vi "Dequeue Message.vi"(8 "error in":errorcluster, 11 "module reference in":T1) -> (0 "error out":errorcluster, 1 "source":T2, 2 "data":variant, 3 "module reference out":T1, 5 "message":T5)   [LabVIEW 2017, in "Logger.lvlib"]
uses:
  Logger.lvlib
  Private TypeDefs/Messages.ctl
  Global TypeDefs/Registered Modules.ctl
  Private TypeDefs/Module Reference.ctl
  Private TypeDefs/Module Queues.ctl
  Private TypeDefs/Message Queue Element.ctl
  Private TypeDefs/Module Notifiers.ctl
  Private TypeDefs/Dummy Notifier.ctl
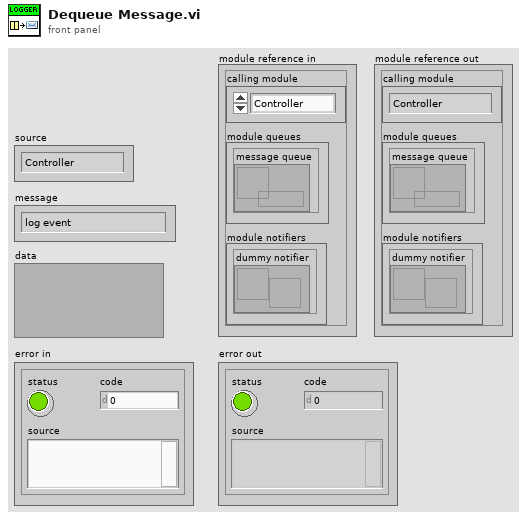
[diagram p1: front panel]
types:
  T1 = typedef "Logger.lvlib/Module Reference.ctl" = cluster{"calling module":T2, "module queues":T3, "module notifiers":T4}
  T2 = typedef "Registered Modules.ctl" = enum16{"Controller", "DAQ", "Error Handler", "Game", "myPAM", "WinHost", "Logger"}
  T3 = typedef "Logger.lvlib/Module Queues.ctl" = cluster{"message queue":refnum<queue>}
  T4 = typedef "Logger.lvlib/Module Notifiers.ctl" = cluster{"dummy notifier":refnum<notifier>}
  T5 = typedef "Logger.lvlib/Messages.ctl" = enum16{"log event", "shutdown"}
  T6 = typedef "Logger.lvlib/Message Queue Element.ctl" = cluster{"source":T2, "message":T5, "data":variant}
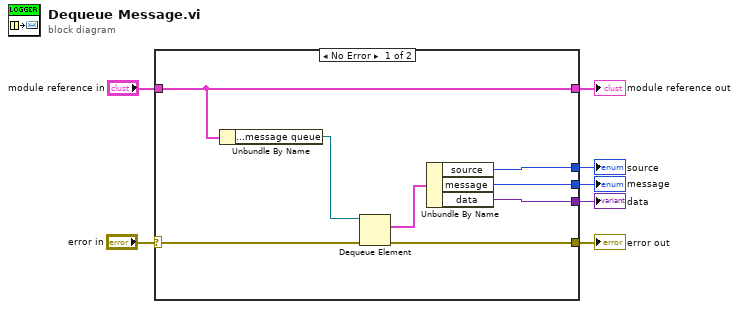
[diagram p0: block diagram]
diagram:
  n1 = case shown="No Error" "error in" {
    selector: "error in" -> [w15 w17]
    tunnel: [w14 w17] -> w6
    tunnel: [w13 _] -> w5
    tunnel: [w12 _] -> w4
    tunnel: "module reference in" -> [w8 w16]
    tunnel: [w9 _] -> w2
    tunnel: [w8 w16] -> w1
    frame No Error {
      n2 = Unbundle By Name(w8) -> ("module queues.message queue"=w10:refnum<queue>)
      n3 = Dequeue Element(queue=w10, error in (no error)=w15) -> (element=w11:T6, error out=w14:errorcluster)  [unwired: 1 in, 2 out]
      n4 = Unbundle By Name(w11) -> ("source"=w9:T2, "message"=w13:T5, "data"=w12:variant)
    }
    frame Error {
    }
  }
  "data" <- w4
  "message" <- w5
  "source" <- w2
  "error out" <- w6
  "module reference out" <- w1
